vi "Get SMO Public API.vi"(8 "error in (no error)":errorcluster, 11 "Instrument.AFM_DLog in":refnum<class "Instrument.AFM_DLog.lvclass">) -> (0 "error out":errorcluster, 2 "Commands":string[](array[string]), 3 "Instrument.AFM_DLog out":refnum<class "Instrument.AFM_DLog.lvclass">)   [LabVIEW 2019, in "Instrument.AFM_DLog.lvclass"]
uses:
  Instrument.AFM_DLog.lvclass
  <userlib>/LevyLab/Instrument Framework/Instrument Types/SCPI/Instrument.SCPI.lvclass
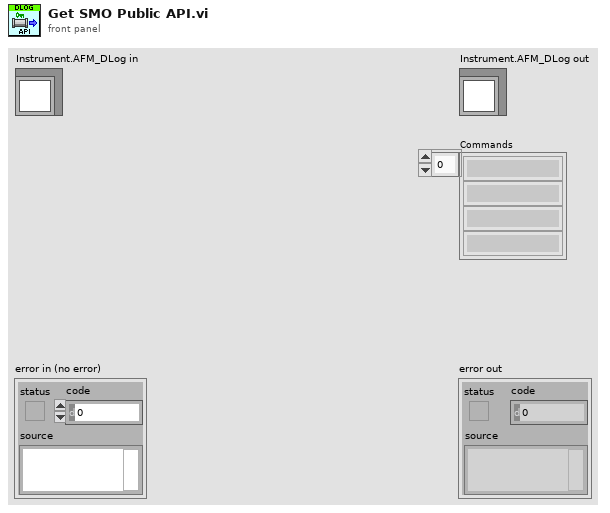
[diagram p1: front panel]
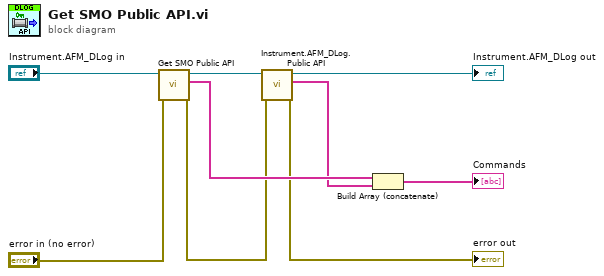
[diagram p0: block diagram]
diagram:
  n1 = call-parent "Get SMO Public API.vi"("error in (no error)"="error in (no error)", "Instrument in"="Instrument.AFM_DLog in") -> ("error out"=w3:errorcluster, "commands"=w8:string[], "Instrument out"=w4:refnum<class "Instrument.AFM_DLog.lvclass">)  [unwired: 7 in]
  n2 = call "Instrument.AFM_DLog.Public API.vi"("error in (no error)"=w3, "Instrument.AFM_DLog in"=w4) -> ("error out"=→"error out":errorcluster, "commands (this level)"=w5:string[], "Instrument.AFM_DLog out"=→"Instrument.AFM_DLog out":refnum<class "Instrument.AFM_DLog.lvclass">)  [unwired: 7 in]
  n3 = Build Array (concatenate)(w8, w5) -> (→"Commands":string[])
